vi "SCMP FITS - Make Single FITS Header coop.vi"(6 "FITS info":T1={"File name"="lsob_demo_0530_LM_20190529_124525_live_C1_00020_001_lev0.0.fits", "Date"="2019-05-29T12:45:25"}, 7 "Camera.lvclass":refnum<class "Camera.lvclass">, 8 "error in":errorcluster, 9 "NAXIS":string="2", 10 "FITS Header":T2={"Wavelength (nm)"=530.15, "Exposure (s)"=0.05, "Tuning Delay (ms)"=1000.0, "Beam Type (-1/1)"=1.0, "Tuning Voltages"=[1.111, 2.222, 3.333, 4.444], "Observer"="observer", "Light Shapping Diffuser"=enum."In Beam", "Comment"="", "Data Type"=enum."HOLE", "Mod Cycles"=0, "SCD Calibration Optics"=enum."1 - Polarizer @0, I+Q", "SCD Emission Line Filter"=enum."1-557.6nm", "Cookbook"="", "COMP-S Calibration Wheel"=enum."Dark", "COMP-S Andover Filter Wheel"=enum."530.3nm/HWB 0.34nm (Fe XIV)", "FOV Rotation (deg)"=66.0, "Objective Lens Position (mm)"=0.0, "Occulter size"=0.0, "Time End"=timestamp(3382374145.421875 s since 1904-01-01), "Acc Exposure (s)"=0.0, "Time Stamp Array"=[], "Camera Serial Number"=[], "Camera Temp"=[], "Camera PI (mm)"=[], "Time Start"=timestamp(3382374145.421875 s since 1904-01-01), "Peripherals"={"ILX controler"=FALSE, "Zone temperatures"=FALSE, "Andor"=FALSE, "Andor 2"=FALSE, "PI Stages"=FALSE, "AISAS mechanisms"=FALSE, "AISAS Mech.lvclass"=refnum, "Zone temp ref"=variant, "FWs"=FALSE}, "FITS paths"=[], "Cameras"=enum."Andor", "load preset cbk"=FALSE, "periodic check count"=0, "COMP-S Calibration Wheel 2"=enum."Dark", "Calib"=enum."Dark", "Abso Aperture"=66.0, "Nominal Aperture"=66.0} {"Nominal Aperture" format="%.1f"; "Abso Aperture" format="%.1f"; "Camera PI (mm)" format="%_3g"; "Acc Exposure (s)" format="%^.3g"; "Occulter size" format="%.2f"; "Objective Lens Position (mm)" min=70.0 max=152.0 format="%.2f"; "FOV Rotation (deg)" format="%.1f"; "Exposure (s)" format="%^.3g"; "Wavelength (nm)" format="%_6g"}, 11 "Image #":i32) -> (0 "error out":errorcluster, 1 "23040 Byte Header":string="SIMPLE  =                              T / CONFORMS TO FITS STANDARD            BITPIX  =                             32 / BITS PER PIXEL                       NAXIS   =                              2 / DATA DIMENSIONS IN FITS FILE         NAXIS1  =                              0 / XDIM (PIXELS)                        NAXIS2  =                              0 / YDIM (PIXELS)                        NAXIS3  =                              4 / 4 POLARIZATION STATES                NAXIS4  =                              1 / 1 CAMERA                             ORIGIN  =                        'AISAS' / SCIENTIFIC GROUP                     OBSERVER=                     'SCHWARTZ' / NAME OF OBSERVER                     TELESCOP=                   '20CM ZEISS' / NAME OF TELESCOPE                    LOCATION=            'LOMNICKY PEAK OBS' / LOCATION OF TELESCOPE                INSTRUME=                          'SCD' / NAME OF INSTRUMENT                   BZERO   =                             0. /  ADU OFFSET                          FOCUS   =                             26 / CAMERA-STAGE POSITION (MM)           ROTPOS  =                           66.0 / ROTATIONAL POSITION (DEG)            DIFFUSER=                      'IN BEAM' / 0=IN BEAM, 1=OUT OF BEAM             FW-WVLNG=                        '557.6' / PRE-FILTER CENTER WAVELENGTH (NM)    FW-CALIB=                         'DARK' / CAL-WHEEL POSITION                   CAM-SN1 =                    'SCC-02209' / CAMERA SERIAL NUMBER                 CAM-TEMP=                       0.000000 / FOCAL PLANE TEMP (C)                 TUNEDLAY=                           1000 / LCVR RELAXATION DELAY (mS)           DATE_OBS=                     '3/7/2011' / DATE OF OBSERVATION START (UTC)      TIME_OBS=                   '212225.421' / TIME OF OBSERVATION (UTC)            EXPOSURE=                       0.050000 / EXPOSURE TIME (S)                    MODC    =                              0 / NUMBER OF IMAGES AT EACH STATE       NLC-1   =                          1.111 / TUNING VOLTAGE-1                     NLC-2   =                          2.222 / TUNING VOLTAGE-2                     NLC-3   =                          3.333 / TUNING VOLTAGE-3                     NLC-4   =                          4.444 / TUNING VOLTAGE-4                     NLC-5   =                          0.000 / TUNING VOLTAGE-5                     BEAM    =                              1 / BEAM (0=ON BAND OR 1=CONTINUUM)      WAVELENG=                         530.15 / WAVELENGTH OF OBS (NM)               COMMHEAD=                             '' / OBSERVER COMMENT                     COOKBOOK=                                / COOKBOOK  LOADED                     COMMENT                                                                         COMMENT                                                                         COMMENT                                                                         COMMENT                                                                         COMMENT                                                                         COMMENT                                                                         COMMENT                                                                         COMMENT                                                                         COMMENT                                                                         COMMENT                                                                         COMMENT                                                                         COMMENT                                                                         COMMENT                                                                         COMMENT                                                                         COMMENT                                                                         COMMENT                                                                         COMMENT                                                                         COMMENT                                                                         COMMENT                                                                         COMMENT                                                                         COMMENT                                                                         COMMENT                                                                         COMMENT                                                                         COMMENT                                                                         COMMENT                                                                         COMMENT                                                                         COMMENT                                                                         COMMENT                                                                         COMMENT                                                                         COMMENT                                                                         COMMENT                                                                         COMMENT                                                                         COMMENT                                                                         COMMENT                                                                         COMMENT                                                                         COMMENT                                                                         COMMENT                                                                         COMMENT                                                                         COMMENT                                                                         COMMENT                                                                         COMMENT                                                                         COMMENT                                                                         COMMENT                                                                         COMMENT                                                                         COMMENT                                                                         COMMENT                                                                         COMMENT                                                                         COMMENT                                                                         COMMENT                                                                         COMMENT                                                                         COMMENT                                                                         COMMENT                                                                         COMMENT                                                                         COMMENT                                                                         COMMENT                                                                         COMMENT                                                                         COMMENT                                                                         COMMENT                                                                         COMMENT                                                                         COMMENT                                                                         COMMENT                                                                         COMMENT                                                                         COMMENT                                                                         COMMENT                                                                         COMMENT                                                                         COMMENT                                                                         COMMENT                                                                         COMMENT                                                                         COMMENT                                                                         COMMENT                                                                         COMMENT                                                                         COMMENT                                                                         COMMENT                                                                         COMMENT                                                                         COMMENT                                                                         COMMENT                                                                         COMMENT                                                                         COMMENT                                                                         COMMENT                                                                         COMMENT                                                                         COMMENT                                                                         COMMENT                                                                         COMMENT                                                                         COMMENT                                                                         COMMENT                                                                         COMMENT                                                                         COMMENT                                                                         COMMENT                                                                         COMMENT                                                                         COMMENT                                                                         COMMENT                                                                         COMMENT                                                                         COMMENT                                                                         COMMENT                                                                         COMMENT                                                                         COMMENT                                                                         COMMENT                                                                         COMMENT                                                                         COMMENT                                                                         COMMENT                                                                         COMMENT                                                                         COMMENT                                                                         COMMENT                                                                         COMMENT                                                                         COMMENT                                                                         COMMENT                                                                         COMMENT                                                                         COMMENT                                                                         COMMENT                                                                         COMMENT                                                                         COMMENT                                                                         COMMENT                                                                         COMMENT                                                                         COMMENT                                                                         COMMENT                                                                         COMMENT                                                                         COMMENT                                                                         COMMENT                                                                         COMMENT                                                                         COMMENT                                                                         COMMENT                                                                         COMMENT                                                                         COMMENT                                                                         COMMENT                                                                         COMMENT                                                                         COMMENT                                                                         COMMENT                                                                         COMMENT                                                                         COMMENT                                                                         COMMENT                                                                         COMMENT                                                                         COMMENT                                                                         COMMENT                                                                         COMMENT                                                                         COMMENT                                                                         COMMENT                                                                         COMMENT                                                                         COMMENT                                                                         COMMENT                                                                         COMMENT                                                                         COMMENT                                                                         COMMENT                                                                         COMMENT                                                                         COMMENT                                                                         COMMENT                                                                         COMMENT                                                                         COMMENT                                                                         COMMENT                                                                         COMMENT                                                                         COMMENT                                                                         COMMENT                                                                         COMMENT                                                                         COMMENT                                                                         COMMENT                                                                         COMMENT                                                                         COMMENT                                                                         COMMENT                                                                         COMMENT                                                                         COMMENT                                                                         COMMENT                                                                         COMMENT                                                                         COMMENT                                                                         COMMENT                                                                         COMMENT                                                                         COMMENT                                                                         COMMENT                                                                         COMMENT                                                                         COMMENT                                                                         COMMENT                                                                         COMMENT                                                                         COMMENT                                                                         COMMENT                                                                         COMMENT                                                                         COMMENT                                                                         COMMENT                                                                         COMMENT                                                                         COMMENT                                                                         COMMENT                                                                         COMMENT                                                                         COMMENT                                                                         COMMENT                                                                         COMMENT                                                                         COMMENT                                                                         COMMENT                                                                         COMMENT                                                                         COMMENT                                                                         COMMENT                                                                         COMMENT                                                                         COMMENT                                                                         COMMENT                                                                         COMMENT                                                                         COMMENT                                                                         COMMENT                                                                         COMMENT                                                                         COMMENT                                                                         COMMENT                                                                         COMMENT                                                                         COMMENT                                                                         COMMENT                                                                         COMMENT                                                                         COMMENT                                                                         COMMENT                                                                         COMMENT                                                                         COMMENT                                                                         COMMENT                                                                         COMMENT                                                                         COMMENT                                                                         COMMENT                                                                         COMMENT                                                                         COMMENT                                                                         COMMENT                                                                         COMMENT                                                                         COMMENT                                                                         COMMENT                                                                         COMMENT                                                                         COMMENT                                                                         COMMENT                                                                         COMMENT                                                                         COMMENT                                                                         COMMENT                                                                         COMMENT                                                                         COMMENT                                                                         COMMENT                                                                         COMMENT                                                                         COMMENT                                                                         COMMENT                                                                         COMMENT                                                                         COMMENT                                                                         COMMENT                                                                         COMMENT                                                                         COMMENT                                                                         COMMENT                                                                         COMMENT                                                                         COMMENT                                                                         COMMENT                                                                         COMMENT                                                                         COMMENT                                                                         COMMENT                                                                         COMMENT                                                                         COMMENT                                                                         COMMENT                                                                         COMMENT                                                                         COMMENT                                                                         COMMENT                                                                         COMMENT                                                                         COMMENT                                                                         COMMENT                                                                         COMMENT                                                                         COMMENT                                                                         COMMENT                                                                         COMMENT                                                                         COMMENT                                                                         COMMENT                                                                         END                                                                             ", 3 "final header byte length":i32=23040)   [LabVIEW 2014]
uses:
  Controls/SCD - FITS Cluster.ctl
  AISAS/Mech/AISAS Mech.lvclass
  AISAS/Controls/Diffuser.ctl
  Controls/FITS Data type.ctl
  Controls/SCD - Calibration Optics Filter Wheel.ctl
  Controls/SCD - EDT - Emission Line Filter Wheel.ctl
  Controls/CoMP-S Controls/Polarization Optics Filter Wheel.ctl
  Controls/CoMP-S Controls/Emission Line Filter Wheel.ctl
  AISAS/Controls/focus.ctl
  Controls/peripherals.ctl
  Controls/Cameras select.ctl
  Controls/Fits info.ctl
  Camera/Camera/Camera.lvclass
  Controls/Globals.vi
panel:
  out "Required COMMENT Rows":i32
  in  "NAXIS2":string="2160"
  in  "NAXIS1":string="2560"
  out "Header Rows":i32=34
  out "FITS Header":string[](array[string])=["SIMPLE  =                              T / CONFORMS TO FITS STANDARD            ", "BITPIX  =                             32 / BITS PER PIXEL                       ", "NAXIS   =                              2 / DATA DIMENSIONS IN FITS FILE         ", "NAXIS1  =                              0 / XDIM (PIXELS)                        ", "NAXIS2  =                              0 / YDIM (PIXELS)                        ", "NAXIS3  =                              4 / 4 POLARIZATION STATES                ", "NAXIS4  =                              1 / 1 CAMERA                             ", "ORIGIN  =                        'AISAS' / SCIENTIFIC GROUP                     ", "OBSERVER=                     'SCHWARTZ' / NAME OF OBSERVER                     ", "TELESCOP=                   '20CM ZEISS' / NAME OF TELESCOPE                    ", "LOCATION=            'LOMNICKY PEAK OBS' / LOCATION OF TELESCOPE                ", "INSTRUME=                          'SCD' / NAME OF INSTRUMENT                   ", "BZERO   =                             0. /  ADU OFFSET                          ", "FOCUS   =                             26 / CAMERA-STAGE POSITION (MM)           ", "ROTPOS  =                           66.0 / ROTATIONAL POSITION (DEG)            ", "DIFFUSER=                      'IN BEAM' / 0=IN BEAM, 1=OUT OF BEAM             ", "FW-WVLNG=                        '557.6' / PRE-FILTER CENTER WAVELENGTH (NM)    ", "FW-CALIB=                         'DARK' / CAL-WHEEL POSITION                   ", "CAM-SN1 =                    'SCC-02209' / CAMERA SERIAL NUMBER                 ", "CAM-TEMP=                       0.000000 / FOCAL PLANE TEMP (C)                 ", "TUNEDLAY=                           1000 / LCVR RELAXATION DELAY (mS)           ", "DATE_OBS=                     '3/7/2011' / DATE OF OBSERVATION START (UTC)      ", "TIME_OBS=                   '212225.421' / TIME OF OBSERVATION (UTC)            ", "EXPOSURE=                       0.050000 / EXPOSURE TIME (S)                    ", "MODC    =                              0 / NUMBER OF IMAGES AT EACH STATE       ", "NLC-1   =                          1.111 / TUNING VOLTAGE-1                     ", "NLC-2   =                          2.222 / TUNING VOLTAGE-2                     ", "NLC-3   =                          3.333 / TUNING VOLTAGE-3                     ", "NLC-4   =                          4.444 / TUNING VOLTAGE-4                     ", "NLC-5   =                          0.000 / TUNING VOLTAGE-5                     ", "BEAM    =                              1 / BEAM (0=ON BAND OR 1=CONTINUUM)      ", "WAVELENG=                         530.15 / WAVELENGTH OF OBS (NM)               ", "COMMHEAD=                             '' / OBSERVER COMMENT                     ", "COOKBOOK=                                / COOKBOOK  LOADED                     ", "COMMENT                                                                         ", "COMMENT                                                                         ", "COMMENT                                                                         ", "COMMENT                                                                         ", "COMMENT                                                                         ", "COMMENT                                                                         ", "COMMENT                                                                         ", "COMMENT                                                                         ", "COMMENT                                                                         ", "COMMENT                                                                         ", "COMMENT                                                                         ", "COMMENT                                                                         ", "COMMENT                                                                         ", "COMMENT                                                                         ", "COMMENT                                                                         ", "COMMENT                                                                         ", "COMMENT                                                                         ", "COMMENT                                                                         ", "COMMENT                                                                         ", "COMMENT                                                                         ", "COMMENT                                                                         ", "COMMENT                                                                         ", "COMMENT                                                                         ", "COMMENT                                                                         ", "COMMENT                                                                         ", "COMMENT                                                                         ", "COMMENT                                                                         ", "COMMENT                                                                         ", "COMMENT                                                                         ", "COMMENT                                                                         ", "COMMENT                                                                         ", "COMMENT                                                                         ", "COMMENT                                                                         ", "COMMENT                                                                         ", "COMMENT                                                                         ", "COMMENT                                                                         ", "COMMENT                                                                         ", "COMMENT                                                                         ", "COMMENT                                                                         ", "COMMENT                                                                         ", "COMMENT                                                                         ", "COMMENT                                                                         ", "COMMENT                                                                         ", "COMMENT                                                                         ", "COMMENT                                                                         ", "COMMENT                                                                         ", "COMMENT                                                                         ", "COMMENT                                                                         ", "COMMENT                                                                         ", "COMMENT                                                                         ", "COMMENT                                                                         ", "COMMENT                                                                         ", "COMMENT                                                                         ", "COMMENT                                                                         ", "COMMENT                                                                         ", "COMMENT                                                                         ", "COMMENT                                                                         ", "COMMENT                                                                         ", "COMMENT                                                                         ", "COMMENT                                                                         ", "COMMENT                                                                         ", "COMMENT                                                                         ", "COMMENT                                                                         ", "COMMENT                                                                         ", "COMMENT                                                                         ", "COMMENT                                                                         ", "COMMENT                                                                         ", "COMMENT                                                                         ", "COMMENT                                                                         ", "COMMENT                                                                         ", "COMMENT                                                                         ", "COMMENT                                                                         ", "COMMENT                                                                         ", "COMMENT                                                                         ", "COMMENT                                                                         ", "COMMENT                                                                         ", "COMMENT                                                                         ", "COMMENT                                                                         ", "COMMENT                                                                         ", "COMMENT                                                                         ", "COMMENT                                                                         ", "COMMENT                                                                         ", "COMMENT                                                                         ", "COMMENT                                                                         ", "COMMENT                                                                         ", "COMMENT                                                                         ", "COMMENT                                                                         ", "COMMENT                                                                         ", "COMMENT                                                                         ", "COMMENT                                                                         ", "COMMENT                                                                         ", "COMMENT                                                                         ", "COMMENT                                                                         ", "COMMENT                                                                         ", "COMMENT                                                                         ", "COMMENT                                                                         ", "COMMENT                                                                         ", "COMMENT                                                                         ", "COMMENT                                                                         ", "COMMENT                                                                         ", "COMMENT                                                                         ", "COMMENT                                                                         ", "COMMENT                                                                         ", "COMMENT                                                                         ", "COMMENT                                                                         ", "COMMENT                                                                         ", "COMMENT                                                                         ", "COMMENT                                                                         ", "COMMENT                                                                         ", "COMMENT                                                                         ", "COMMENT                                                                         ", "COMMENT                                                                         ", "COMMENT                                                                         ", "COMMENT                                                                         ", "COMMENT                                                                         ", "COMMENT                                                                         ", "COMMENT                                                                         ", "COMMENT                                                                         ", "COMMENT                                                                         ", "COMMENT                                                                         ", "COMMENT                                                                         ", "COMMENT                                                                         ", "COMMENT                                                                         ", "COMMENT                                                                         ", "COMMENT                                                                         ", "COMMENT                                                                         ", "COMMENT                                                                         ", "COMMENT                                                                         ", "COMMENT                                                                         ", "COMMENT                                                                         ", "COMMENT                                                                         ", "COMMENT                                                                         ", "COMMENT                                                                         ", "COMMENT                                                                         ", "COMMENT                                                                         ", "COMMENT                                                                         ", "COMMENT                                                                         ", "COMMENT                                                                         ", "COMMENT                                                                         ", "COMMENT                                                                         ", "COMMENT                                                                         ", "COMMENT                                                                         ", "COMMENT                                                                         ", "COMMENT                                                                         ", "COMMENT                                                                         ", "COMMENT                                                                         ", "COMMENT                                                                         ", "COMMENT                                                                         ", "COMMENT                                                                         ", "COMMENT                                                                         ", "COMMENT                                                                         ", "COMMENT                                                                         ", "COMMENT                                                                         ", "COMMENT                                                                         ", "COMMENT                                                                         ", "COMMENT                                                                         ", "COMMENT                                                                         ", "COMMENT                                                                         ", "COMMENT                                                                         ", "COMMENT                                                                         ", "COMMENT                                                                         ", "COMMENT                                                                         ", "COMMENT                                                                         ", "COMMENT                                                                         ", "COMMENT                                                                         ", "COMMENT                                                                         ", "COMMENT                                                                         ", "COMMENT                                                                         ", "COMMENT                                                                         ", "COMMENT                                                                         ", "COMMENT                                                                         ", "COMMENT                                                                         ", "COMMENT                                                                         ", "COMMENT                                                                         ", "COMMENT                                                                         ", "COMMENT                                                                         ", "COMMENT                                                                         ", "COMMENT                                                                         ", "COMMENT                                                                         ", "COMMENT                                                                         ", "COMMENT                                                                         ", "COMMENT                                                                         ", "COMMENT                                                                         ", "COMMENT                                                                         ", "COMMENT                                                                         ", "COMMENT                                                                         ", "COMMENT                                                                         ", "COMMENT                                                                         ", "COMMENT                                                                         ", "COMMENT                                                                         ", "COMMENT                                                                         ", "COMMENT                                                                         ", "COMMENT                                                                         ", "COMMENT                                                                         ", "COMMENT                                                                         ", "COMMENT                                                                         ", "COMMENT                                                                         ", "COMMENT                                                                         ", "COMMENT                                                                         ", "COMMENT                                                                         ", "COMMENT                                                                         ", "COMMENT                                                                         ", "COMMENT                                                                         ", "COMMENT                                                                         ", "COMMENT                                                                         ", "COMMENT                                                                         ", "COMMENT                                                                         ", "COMMENT                                                                         ", "COMMENT                                                                         ", "COMMENT                                                                         ", "COMMENT                                                                         ", "COMMENT                                                                         ", "COMMENT                                                                         ", "COMMENT                                                                         ", "COMMENT                                                                         ", "COMMENT                                                                         ", "COMMENT                                                                         ", "COMMENT                                                                         ", "COMMENT                                                                         ", "COMMENT                                                                         ", "COMMENT                                                                         ", "COMMENT                                                                         ", "COMMENT                                                                         ", "COMMENT                                                                         ", "COMMENT                                                                         ", "COMMENT                                                                         ", "COMMENT                                                                         ", "COMMENT                                                                         ", "COMMENT                                                                         ", "COMMENT                                                                         ", "COMMENT                                                                         ", "COMMENT                                                                         ", "COMMENT                                                                         ", "COMMENT                                                                         ", "COMMENT                                                                         ", "COMMENT                                                                         ", "COMMENT                                                                         ", "COMMENT                                                                         ", "COMMENT                                                                         ", "COMMENT                                                                         ", "COMMENT                                                                         ", "COMMENT                                                                         ", "COMMENT                                                                         ", "COMMENT                                                                         ", "COMMENT                                                                         ", "COMMENT                                                                         ", "COMMENT                                                                         ", "COMMENT                                                                         ", "COMMENT                                                                         ", "COMMENT                                                                         ", "COMMENT                                                                         ", "COMMENT                                                                         ", "COMMENT                                                                         ", "END                                                                             "]
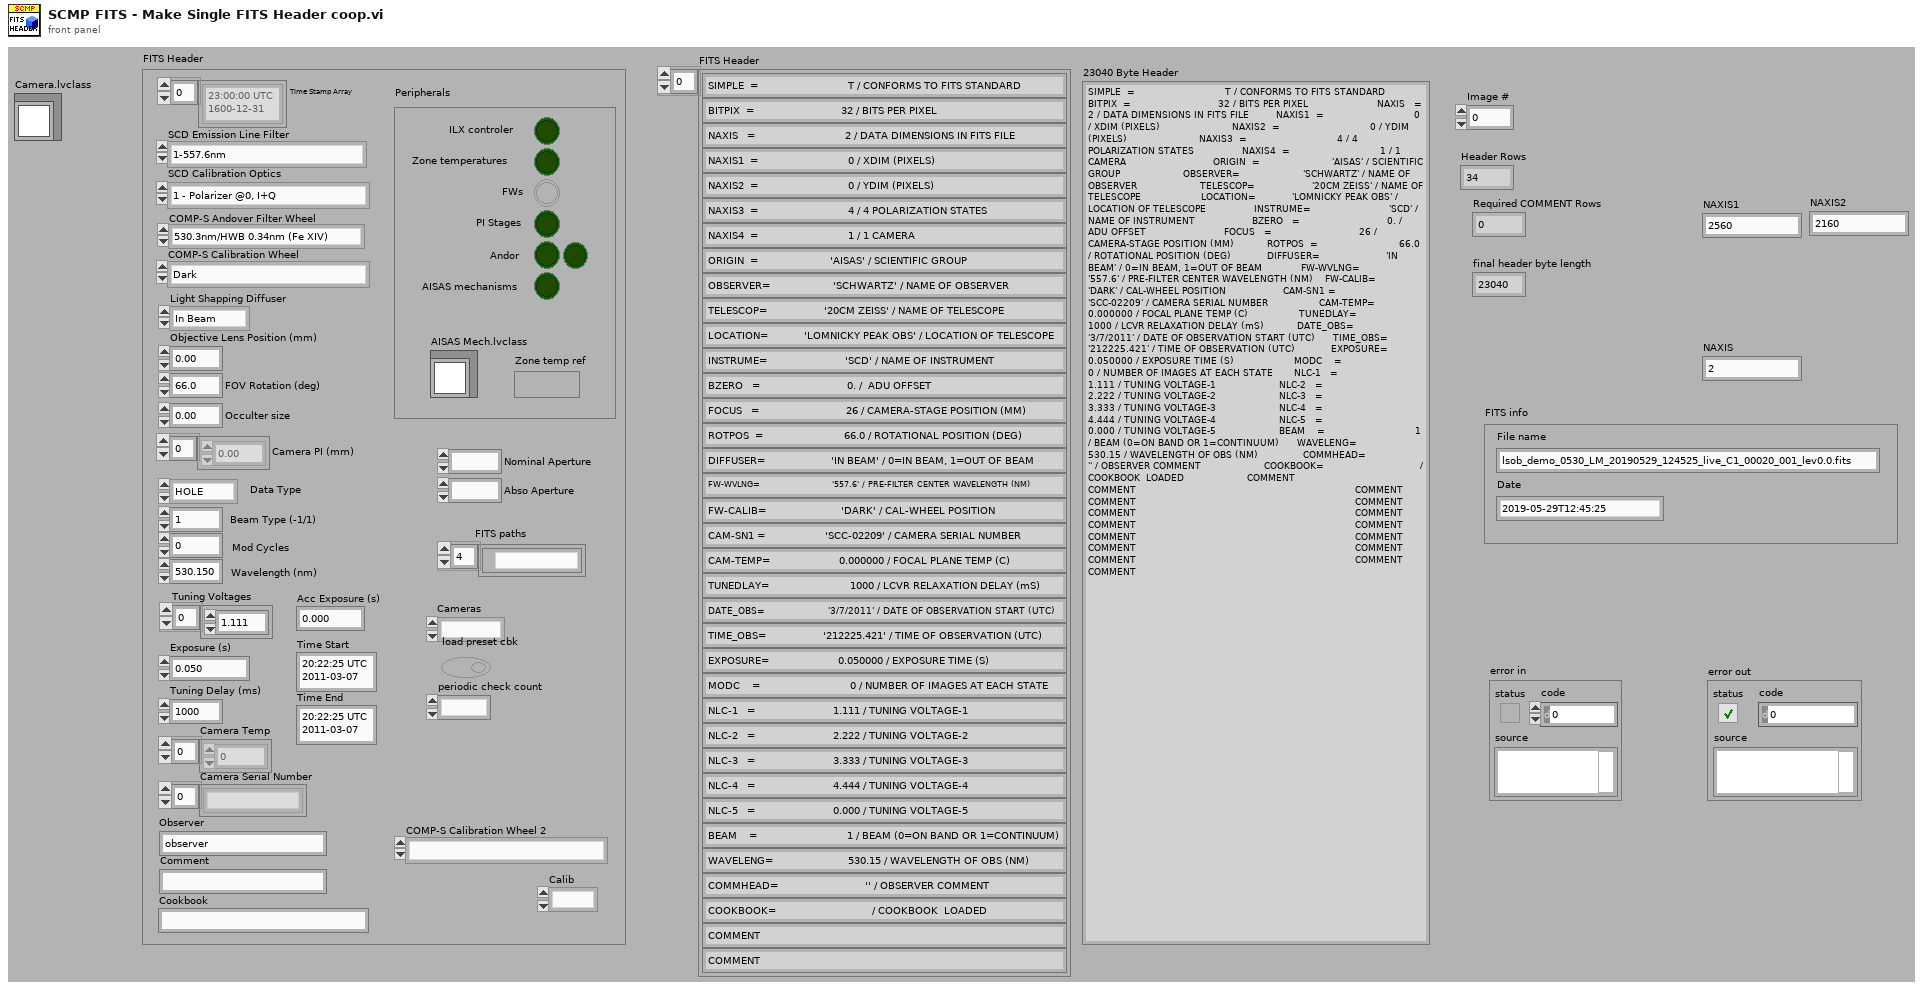
[diagram p1: front panel]
types:
  T1 = typedef "Fits info.ctl" = cluster{"File name":string, "Date":string}
  T2 = typedef "SCD - FITS Cluster.ctl" = cluster{"Wavelength (nm)":dbl, "Exposure (s)":dbl, "Tuning Delay (ms)":dbl, "Beam Type (-1/1)":dbl, "Tuning Voltages":dbl[], "Observer":string, "Light Shapping Diffuser":T3, "Comment":string, "Data Type":T4, "Mod Cycles":u16, "SCD Calibration Optics":T5, "SCD Emission Line Filter":T6, "Cookbook":string, "COMP-S Calibration Wheel":T7, "COMP-S Andover Filter Wheel":T8, "FOV Rotation (deg)":dbl, "Objective Lens Position (mm)":T9, "Occulter size":dbl, "Time End":timestamp, "Acc Exposure (s)":dbl, "Time Stamp Array":timestamp[], "Camera Serial Number":string[], "Camera Temp":dbl[], "Camera PI (mm)":dbl[], "Time Start":timestamp, "Peripherals":T10, "FITS paths":path[], "Cameras":T11, "load preset cbk":bool, "periodic check count":i32, "COMP-S Calibration Wheel 2":T7, "Calib":enum16{"Dark", "Flat"}, "Abso Aperture":dbl, "Nominal Aperture":dbl}
  T3 = typedef "Diffuser.ctl" = enum16{"Out of Beam", "In Beam"}
  T4 = typedef "FITS Data type.ctl" = enum16{"LIVE", "DARK", "FLAT", "CALI", "OBSE", "ABSO", "AURE", "TARG", "OBJE", "HOLE", "OREX", "THRO", "CHIP"}
  T5 = typedef "SCD - Calibration Optics Filter Wheel.ctl" = enum16{"1 - Polarizer @0, I+Q", "2 - Polarizer @90, I-Q", "3 - Polarizer @45, I+U", "4 - Polarizer @135, I-U", "5 - Polarizer @0, Retarder @45, I+V", "6 - Polarizer @0, Retarder @135, I-V", "7 - Dark", "8 - Clear", "9 - N/A"}
  T6 = typedef "SCD - EDT - Emission Line Filter Wheel.ctl" = enum16{"1-557.6nm", "2-587.6nm", "3-589.6nm", "4-630.2nm", "5-656.4nm", "6-849.8nm", "7-854.2nm", "8-866.2nm", "9-1083.0nm"}
  T7 = typedef "Polarization Optics Filter Wheel.ctl" = enum16{"Dark", "Clear", "Exchange Lens", "Polarizer @0, I+Q", "Polarizer @90, I-Q", "Polarizer @45, I+U", "Polarizer @135, I-U", "Polarizer @0, Retarder @45, I+V", "Polarizer @0, Retarder @135, I-V"}
  T8 = typedef "Emission Line Filter Wheel.ctl" = enum16{"530.3nm/HWB 0.34nm (Fe XIV)", "587.6nm/HBW 0.44nm (He I D3)", "637.5nm/HBW 0.53nm (Fe X)", "656.3nm/HBW 0.57nm (H-Alpha)", "789.2nm/HBW 0.85nm (Fe XI)", "854.2nm/HBW 1.01nm (Ca I)", "1074.7nm/HBW 2.34nm (Fe XIII)", "1079.8nm/HBW 1.64nm (Fe XIII)", "1083.0nm/HBW 1.66nm (He I)"}
  T9 = typedef "focus.ctl" = dbl
  T10 = typedef "peripherals.ctl" = cluster{"ILX controler":bool, "Zone temperatures":bool, "Andor":bool, "Andor 2":bool, "PI Stages":bool, "AISAS mechanisms":bool, "AISAS Mech.lvclass":refnum<class "AISAS Mech.lvclass">, "Zone temp ref":variant, "FWs":bool}
  T11 = typedef "Cameras select.ctl" = enum16{"Andor", "GDR"}
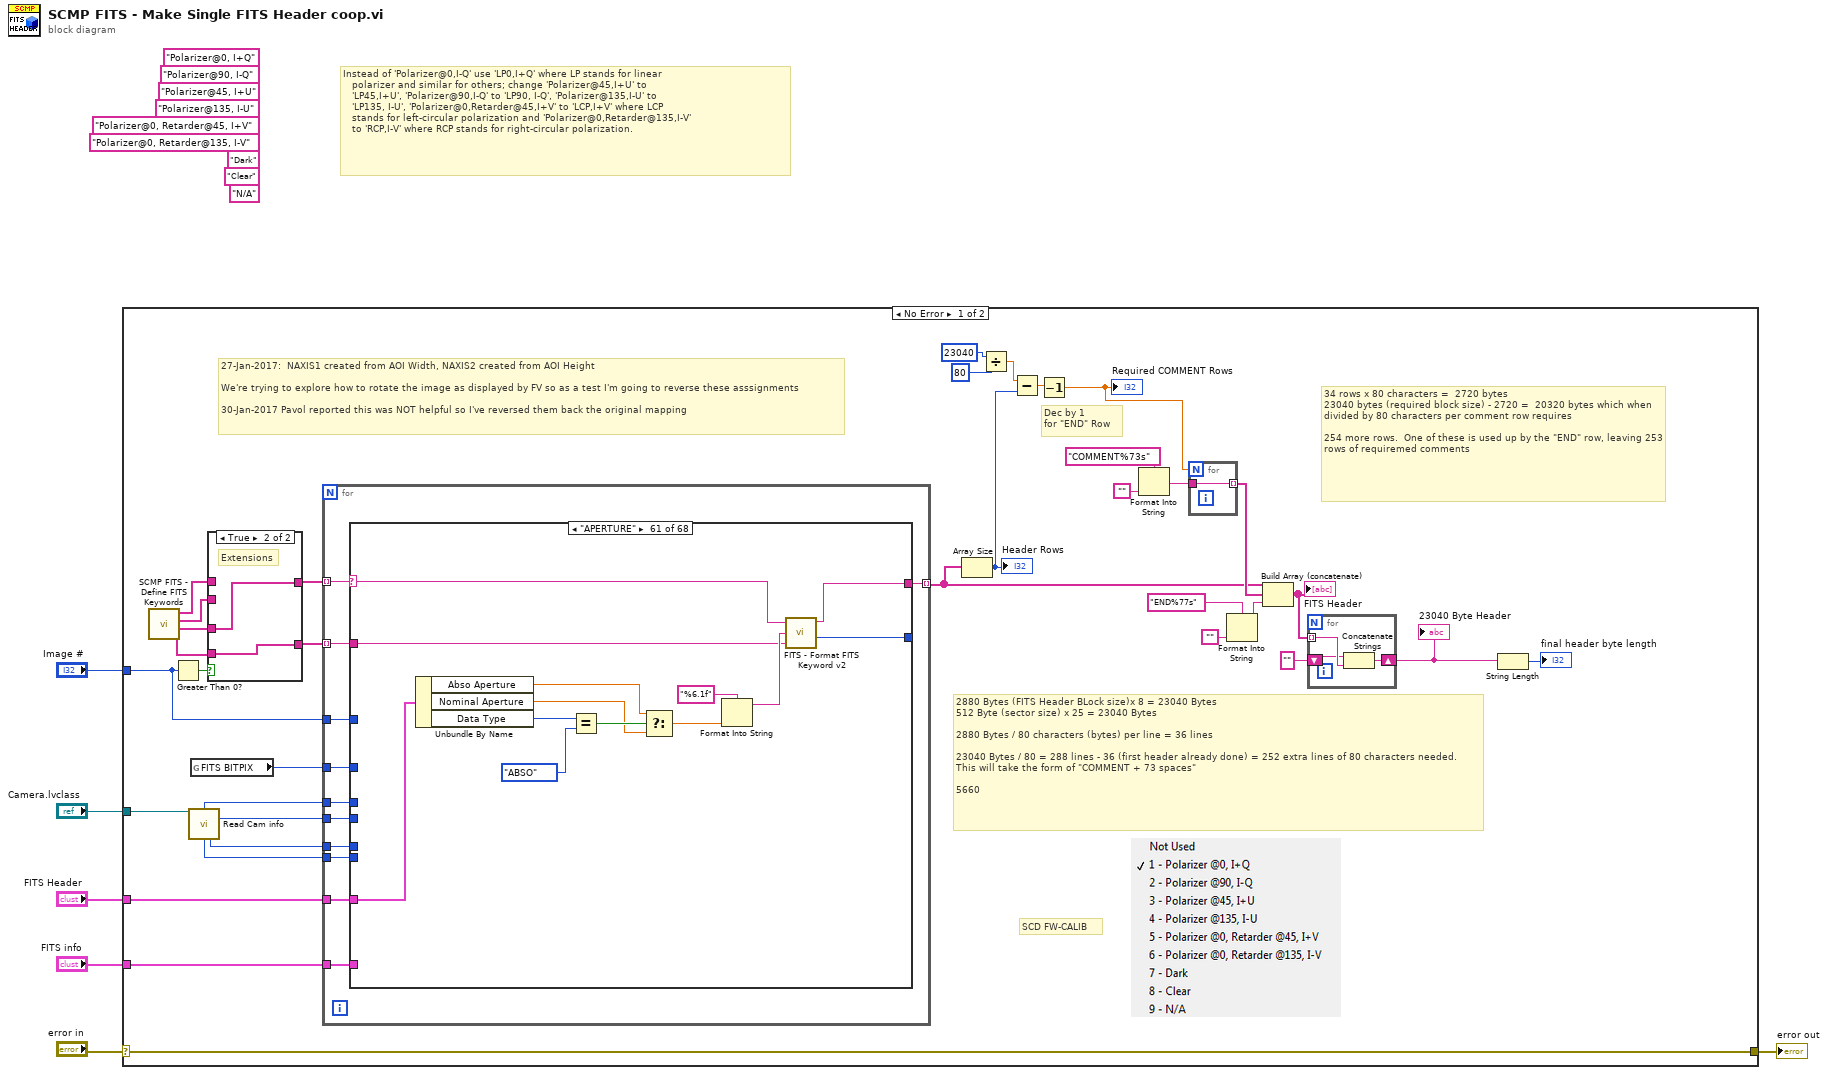
[diagram p0: block diagram]
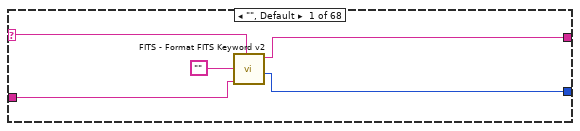
[diagram p3: hidden frame]
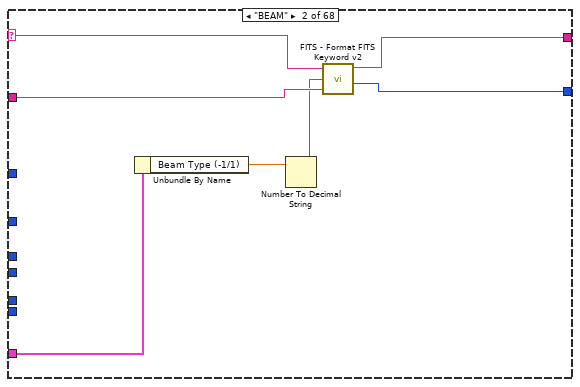
[diagram p4: hidden frame]
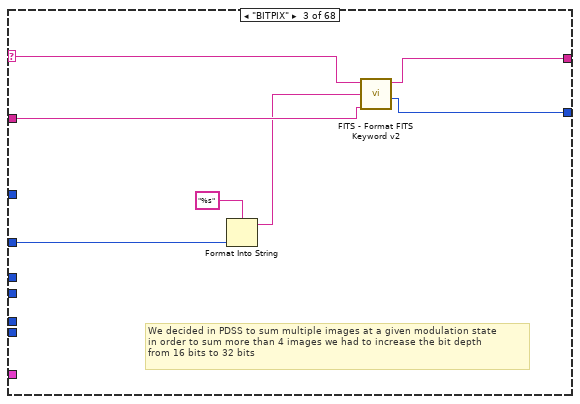
[diagram p5: hidden frame]
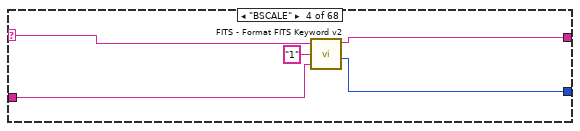
[diagram p6: hidden frame]
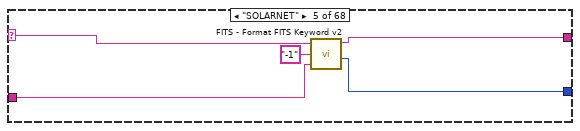
[diagram p7: hidden frame]
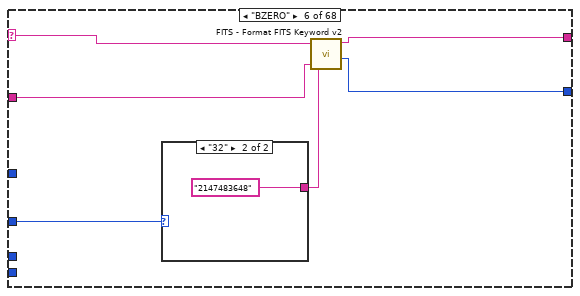
[diagram p8: hidden frame]
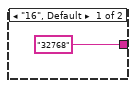
[diagram p9: hidden frame]
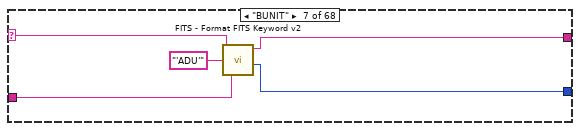
[diagram p10: hidden frame]
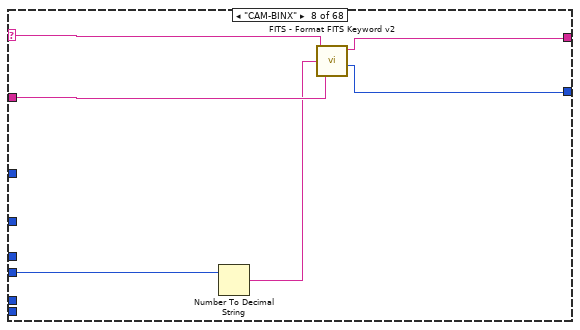
[diagram p11: hidden frame]
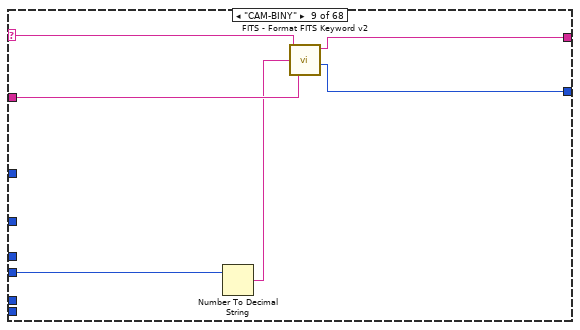
[diagram p12: hidden frame]
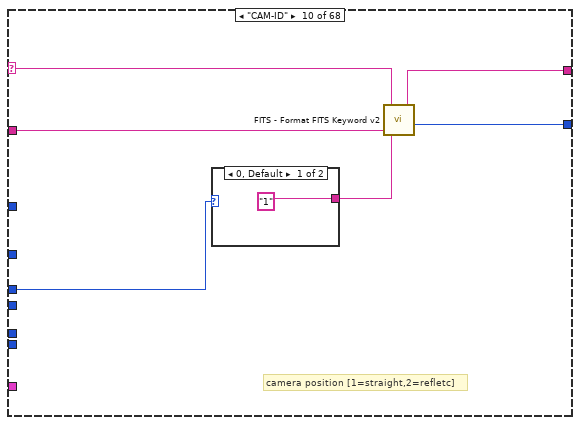
[diagram p13: hidden frame]
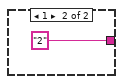
[diagram p14: hidden frame]
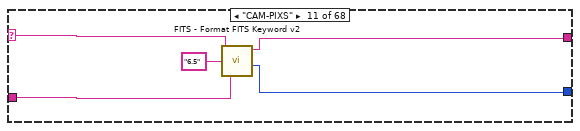
[diagram p15: hidden frame]
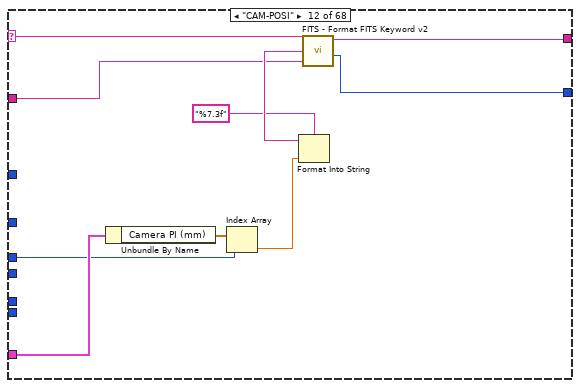
[diagram p16: hidden frame]
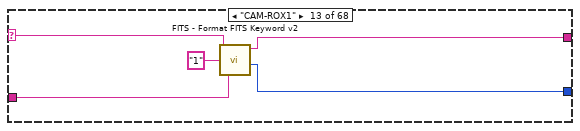
[diagram p17: hidden frame]
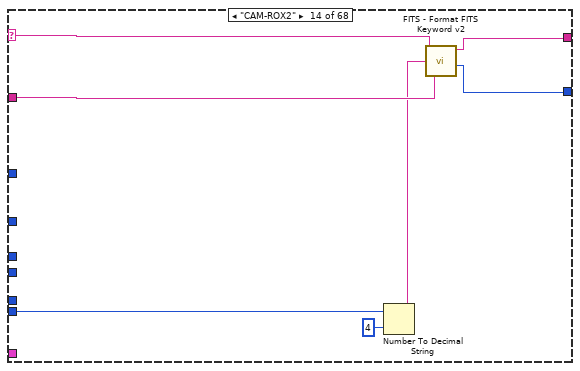
[diagram p18: hidden frame]
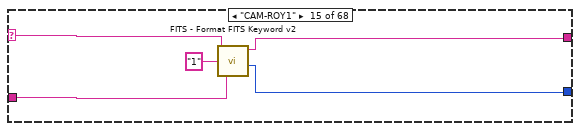
[diagram p19: hidden frame]
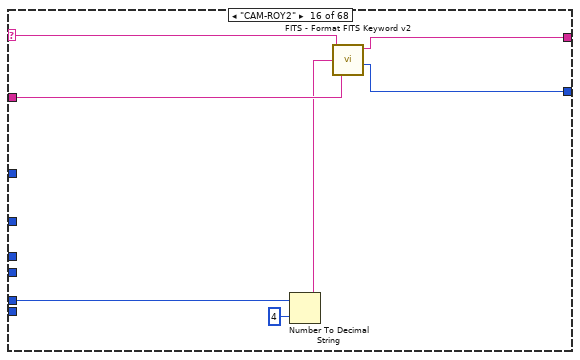
[diagram p20: hidden frame]
diagram:
  (unwired) "N/A" ("element")
  (unwired) "Clear" ("element")
  (unwired) "Dark" ("element")
  (unwired) "Polarizer@0, Retarder@135, I-V" ("element")
  (unwired) "Polarizer@0, Retarder@45, I+V" ("element")
  (unwired) "Polarizer@135, I-U" ("element")
  (unwired) "Polarizer@45, I+U"
  (unwired) "Polarizer@90, I-Q"
  (unwired) "Polarizer@0, I+Q"
  # "Instead of 'Polarizer@0,I-Q' use 'LP0,I+Q' where LP stands for linear\n   polarizer and similar for others; change 'Polarizer@45,I+U' to\n   'LP45,I+U', 'Polarizer@90,I-Q' to 'LP90, I-Q', 'Polarizer@135,I-U' to\n   'LP135, I-U', 'Polarizer@0,Retarder@45,I+V' to 'LCP,I+V' where LCP\n   stands for left-circular polarization and 'Polarizer@0,Retarder@135,I-V'\n   to 'RCP,I-V' where RCP stands for right-circular polarization."
  n1 = case shown="No Error" "error in" {
    selector: "error in" -> [w23 w622]
    tunnel: [w23 w622] -> w5
    tunnel: "Image #" -> [w14 _]
    tunnel: "Camera.lvclass" -> [w12 _]
    tunnel: "FITS Header" -> [w8 _]
    tunnel: "FITS info" -> [w7 _]
    frame No Error {
      # "SCD FW-CALIB"
      # "27-Jan-2017:  NAXIS1 created from AOI Width, NAXIS2 created from AOI Height\n\nWe're trying to explore how to rotate the image as displayed by FV so as a test I'm going to reverse these asssignments\n\n30-Jan-2017 Pavol reported this was NOT helpful so I've reversed them back the original mapping"
      # "34 rows x 80 characters =  2720 bytes\n23040 bytes (required block size) - 2720 =  20320 bytes which when divided by 80 characters per comment row requires\n\n254 more rows.  One of these is used up by the \"END\" row, leaving 253 rows of requiremed comments"
      # "Dec by 1\nfor \"END\" Row"
      # "2880 Bytes (FITS Header BLock size)x 8 = 23040 Bytes\n512 Byte (sector size) x 25 = 23040 Bytes\n\n2880 Bytes / 80 characters (bytes) per line = 36 lines\n\n23040 Bytes / 80 = 288 lines - 36 (first header already done) = 252 extra lines of 80 characters needed.\nThis will take the form of \"COMMENT + 73 spaces\" \n\n5660"
      n2 = call "SCMP FITS - Define FITS Keywords.vi"() -> ("Extension Comments"=w34:string[], "Extension  Keywords"=w35:string[], "Primary Comments"=w36:string[], "Primary Keywords"=w33:string[])  [unwired: 5 in, 3 out]
      n3 = Greater Than 0?(x=w14) -> (x > 0?=w39:bool)
      n4 = call-dynamic "Read Cam info.vi"("Camera in"=w12) -> ("Idx"=w11:i32, "BDiv"=w13:u8, "AOI Width"=w10:i32, "AOI Height"=w9:i32)  [unwired: 5 in, 6 out]
      n5 = global read "Globals.vi" "FITS BITPIX"() -> (w15:enum16{"16", "32"})
      n6 = case shown="True" w39 {
        tunnel: [w47 w49] -> w38
        tunnel: [w46 w48] -> w37
        tunnel: w33 -> [w47 _]
        tunnel: w36 -> [w46 _]
        tunnel: w35 -> [_ w49]
        tunnel: w34 -> [_ w48]
        frame False {
          # "Primary"
        }
        frame True {
          # "Extensions"
        }
      }
      n7 = for {
        tunnel: w38 -> [w56] mode=indexing
        tunnel: w37 -> [w59] mode=indexing
        tunnel: w8 -> [w60]
        tunnel: [w58] -> w22 mode=indexing
        tunnel: w14 -> [w57]
        tunnel: w15 -> [w55]
        tunnel: w7 -> [w54]
        tunnel: w13 -> [w53]
        tunnel: w11 -> [w52]
        tunnel: w10 -> [w51]
        tunnel: w9 -> [w50]
        n8 = case shown="\"APERTURE\"" w56 {
          selector: w56 -> [w65 w72 w79 w84 w89 w95 w101 w108 w114 w120 w126 w135 w141 w149 w153 w161 w171 w181 w187 w194 w202 w226 w233 w248 w260 w266 w274 w284 w295 w306 w316 w321 w329 w334 w341 w345 w353 w362 w394 w399 w404 w411 w415 w422 w430 w449 w456 w467 w472 w482 w492 w502 w512 w522 w530 w538 w545 w551 w556 w560 w574 w582 w587 w591 w597 w608 w613 w620]
          tunnel: w60 -> [_ w69 _ _ _ _ _ _ _ _ _ w130 _ _ _ _ w168 w175 w183 w195 w203 _ w230 w250 w258 w264 w276 w282 _ w303 w313 _ _ _ _ _ w350 w359 w390 _ _ _ _ w419 _ _ _ _ _ w479 w489 w499 w509 w519 w526 w536 w542 _ _ w564 w577 _ _ _ w594 w605 _ w616]
          tunnel: w59 -> [w63 w71 w78 w83 w88 w94 w100 w107 w113 w119 w125 w134 w140 w148 w152 w160 w170 w180 w186 w193 w201 w225 w232 w249 w259 w265 w275 w283 w294 w305 w315 w320 w328 w333 w340 w344 w352 w361 w393 w397 w403 w409 w414 w421 w429 w448 w457 w466 w471 w481 w491 w501 w511 w521 w529 w537 w544 w550 w554 w561 w575 w581 w586 w590 w596 w607 w612 w619]
          tunnel: [w62 w70 w77 w82 w87 w93 w98 w106 w112 w118 w124 w133 w139 w147 w151 w159 w169 w179 w185 w192 w200 w224 w231 w246 w257 w263 w273 w285 w293 w304 w314 w319 w327 w332 w338 w343 w351 w360 w392 w396 w402 w410 w413 w420 w428 w447 w455 w465 w470 w480 w490 w500 w510 w520 w528 w534 w543 w549 w553 w559 w573 w580 w585 w589 w595 w606 w611 w618] -> w58
          tunnel: [w61 w66 w76 w81 w86 w92 w99 w105 w111 w117 w123 w132 w138 w146 w150 w158 w167 w177 w184 w191 w199 w223 w228 w247 w256 w262 w272 w286 w292 w302 w310 w317 w326 w331 w339 w342 w348 w358 w391 w395 w401 w408 w412 w417 w427 w446 w454 w464 w468 w478 w488 w498 w508 w518 w527 w535 w540 w548 w552 w558 w572 w578 w584 w588 w593 w601 w609 w617] -> _
          tunnel: w57 -> [_ _ _ _ _ _ _ _ _ _ _ _ _ _ _ _ _ _ _ _ _ _ _ _ _ _ _ _ _ _ _ _ _ _ _ _ _ _ _ _ _ _ _ _ w425 _ _ _ _ _ _ _ _ _ _ _ _ _ _ _ _ _ _ _ _ _ _ _]
          tunnel: w55 -> [_ _ w75 _ _ w90 _ _ _ _ _ _ _ _ _ _ _ _ _ _ _ _ _ _ _ _ _ _ _ _ _ _ _ _ _ _ _ _ _ _ _ _ _ _ _ _ _ _ _ _ _ _ _ _ _ _ _ _ _ _ _ _ _ _ _ _ _ _]
          tunnel: w54 -> [_ _ _ _ _ _ _ _ _ _ _ _ _ _ _ _ _ _ _ _ _ w221 w227 _ _ _ _ _ _ _ _ _ w325 _ _ _ _ _ _ _ _ _ _ _ _ _ _ _ _ _ _ _ _ _ _ _ _ _ _ _ _ _ _ _ _ _ _ _]
          tunnel: w53 -> [_ _ _ _ _ _ _ w103 w109 _ _ _ _ _ _ _ _ _ _ _ _ _ _ _ _ _ _ _ _ _ _ _ _ _ _ _ _ _ _ _ _ _ _ _ _ _ _ _ _ _ _ _ _ _ _ _ _ _ _ _ _ _ _ _ _ _ _ _]
          tunnel: w52 -> [_ _ _ _ _ _ _ _ _ w115 _ w128 _ _ _ _ w162 w172 _ _ _ _ _ _ _ _ _ _ _ _ _ _ _ _ _ _ _ _ _ _ _ _ _ _ _ _ _ _ _ _ _ _ _ _ _ _ _ _ _ _ _ _ _ _ _ _ _ _]
          tunnel: w51 -> [_ _ _ _ _ _ _ _ _ _ _ _ _ w143 _ _ _ _ _ _ _ _ _ _ _ _ _ _ _ _ _ _ _ _ _ _ _ _ _ _ _ _ _ _ _ w442 w452 _ _ _ _ _ _ _ _ _ _ _ _ _ _ _ _ _ _ _ _ _]
          tunnel: w50 -> [_ _ _ _ _ _ _ _ _ _ _ _ _ _ _ w155 _ _ _ _ _ _ _ _ _ _ _ _ _ _ _ _ _ _ _ _ _ _ _ _ _ _ _ _ _ w441 w453 _ _ _ _ _ _ _ _ _ _ _ _ _ _ _ _ _ _ _ _ _]
          frame "", Default {
            n9 = call "FITS - Format FITS Keyword v2 .vi"("Keyword"=w65, "Value"="", "Comment"=w63) -> ("Formatted fits entry"=w62:string, "Length of line"=w61:i16)  [unwired: 1 in, 1 out]
          }
          frame "BEAM" {
            n10 = Unbundle By Name(w69) -> ("Beam Type (-1/1)"=w67:dbl)
            n11 = Number To Decimal String(number=w67) -> (decimal integer string=w68:string)  [unwired: 1 out]
            n12 = call "FITS - Format FITS Keyword v2 .vi"("Keyword"=w72, "Value"=w68, "Comment"=w71) -> ("Formatted fits entry"=w70:string, "Length of line"=w66:i16)  [unwired: 1 in, 1 out]
          }
          frame "BITPIX" {
            # "We decided in PDSS to sum multiple images at a given modulation state\nin order to sum more than 4 images we had to increase the bit depth\nfrom 16 bits to 32 bits"
            n13 = Format Into String(format string="%s", w75) -> (resulting string=w73:string)  [unwired: 2 in, 1 out]
            n14 = call "FITS - Format FITS Keyword v2 .vi"("Keyword"=w79, "Value"=w73, "Comment"=w78) -> ("Formatted fits entry"=w77:string, "Length of line"=w76:i16)  [unwired: 1 in, 1 out]
          }
          frame "BSCALE" {
            n15 = call "FITS - Format FITS Keyword v2 .vi"("Keyword"=w84, "Value"="1", "Comment"=w83) -> ("Formatted fits entry"=w82:string, "Length of line"=w81:i16)  [unwired: 1 in, 1 out]
          }
          frame "SOLARNET" {
            n16 = call "FITS - Format FITS Keyword v2 .vi"("Keyword"=w89, "Value"="-1", "Comment"=w88) -> ("Formatted fits entry"=w87:string, "Length of line"=w86:i16)  [unwired: 1 in, 1 out]
          }
          frame "BZERO" {
            n17 = case shown="\"32\"" w90 {
              tunnel: ["32768" ("Value") "2147483648" ("Value")] -> w91
              frame "16", Default {
              }
              frame "32" {
              }
            }
            n18 = call "FITS - Format FITS Keyword v2 .vi"("Keyword"=w95, "Value"=w91, "Comment"=w94) -> ("Formatted fits entry"=w93:string, "Length of line"=w92:i16)  [unwired: 1 in, 1 out]
          }
          frame "BUNIT" {
            n19 = call "FITS - Format FITS Keyword v2 .vi"("Keyword"=w101, "Value"="'ADU'", "Comment"=w100) -> ("Formatted fits entry"=w98:string, "Length of line"=w99:i16)  [unwired: 1 in, 1 out]
          }
          frame "CAM-BINX" {
            n20 = Number To Decimal String(number=w103) -> (decimal integer string=w104:string)  [unwired: 1 in]
            n21 = call "FITS - Format FITS Keyword v2 .vi"("Keyword"=w108, "Value"=w104, "Comment"=w107) -> ("Formatted fits entry"=w106:string, "Length of line"=w105:i16)  [unwired: 1 in, 1 out]
          }
          frame "CAM-BINY" {
            n22 = Number To Decimal String(number=w109) -> (decimal integer string=w110:string)  [unwired: 1 in]
            n23 = call "FITS - Format FITS Keyword v2 .vi"("Keyword"=w114, "Value"=w110, "Comment"=w113) -> ("Formatted fits entry"=w112:string, "Length of line"=w111:i16)  [unwired: 1 in, 1 out]
          }
          frame "CAM-ID" {
            # "camera position [1=straight,2=refletc]"
            n24 = case shown="0, Default" w115 {
              tunnel: ["1" ("string") "2" ("string")] -> w116
              frame 0, Default {
              }
              frame 1 {
              }
            }
            n25 = call "FITS - Format FITS Keyword v2 .vi"("Keyword"=w120, "Value"=w116, "Comment"=w119) -> ("Formatted fits entry"=w118:string, "Length of line"=w117:i16)  [unwired: 1 in, 1 out]
          }
          frame "CAM-PIXS" {
            n26 = call "FITS - Format FITS Keyword v2 .vi"("Keyword"=w126, "Value"="6.5", "Comment"=w125) -> ("Formatted fits entry"=w124:string, "Length of line"=w123:i16)  [unwired: 1 in, 1 out]
          }
          frame "CAM-POSI" {
            n27 = Unbundle By Name(w130) -> ("Camera PI (mm)"=w131:dbl[])
            n28 = Index Array(array=w131, index=w128) -> (element=w129:dbl)
            n29 = Format Into String(format string="%7.3f", w129) -> (resulting string=w137:string)  [unwired: 2 in, 1 out]
            n30 = call "FITS - Format FITS Keyword v2 .vi"("Keyword"=w135, "Value"=w137, "Comment"=w134) -> ("Formatted fits entry"=w133:string, "Length of line"=w132:i16)  [unwired: 1 in, 1 out]
          }
          frame "CAM-ROX1" {
            n31 = call "FITS - Format FITS Keyword v2 .vi"("Keyword"=w141, "Value"="1", "Comment"=w140) -> ("Formatted fits entry"=w139:string, "Length of line"=w138:i16)  [unwired: 1 in, 1 out]
          }
          frame "CAM-ROX2" {
            n32 = Number To Decimal String(number=w143, width (-)=i16 4) -> (decimal integer string=w144:string)
            n33 = call "FITS - Format FITS Keyword v2 .vi"("Keyword"=w149, "Value"=w144, "Comment"=w148) -> ("Formatted fits entry"=w147:string, "Length of line"=w146:i16)  [unwired: 1 in, 1 out]
          }
          frame "CAM-ROY1" {
            n34 = call "FITS - Format FITS Keyword v2 .vi"("Keyword"=w153, "Value"="1", "Comment"=w152) -> ("Formatted fits entry"=w151:string, "Length of line"=w150:i16)  [unwired: 1 in, 1 out]
          }
          frame "CAM-ROY2" {
            n35 = Number To Decimal String(number=w155, width (-)=i16 4) -> (decimal integer string=w156:string)
            n36 = call "FITS - Format FITS Keyword v2 .vi"("Keyword"=w161, "Value"=w156, "Comment"=w160) -> ("Formatted fits entry"=w159:string, "Length of line"=w158:i16)  [unwired: 1 in, 1 out]
          }
          frame "CAM-SN" {
            w166 = "'" ("string")
            n37 = Unbundle By Name(w168) -> ("Camera Serial Number"=w164:string[])
            n38 = Index Array(array=w164, index=w162) -> (element=w163:string)
            n39 = Concatenate Strings(w166, w163, w166) -> (w165:string)
            n40 = call "FITS - Format FITS Keyword v2 .vi"("Keyword"=w171, "Value"=w165, "Comment"=w170) -> ("Formatted fits entry"=w169:string, "Length of line"=w167:i16)  [unwired: 1 in, 1 out]
          }
          frame "CAM-TEMP" {
            n41 = Unbundle By Name(w175) -> ("Camera Temp"=w174:dbl[])
            n42 = Index Array(array=w174, index=w172) -> (element=w173:dbl)
            n43 = Format Into String(format string="%6.2f", w173) -> (resulting string=w178:string)  [unwired: 2 in, 1 out]
            n44 = call "FITS - Format FITS Keyword v2 .vi"("Keyword"=w181, "Value"=w178, "Comment"=w180) -> ("Formatted fits entry"=w179:string, "Length of line"=w177:i16)  [unwired: 1 in, 1 out]
          }
          frame "COMMHEAD" {
            n45 = Unbundle By Name(w183) -> ("Comment"=w182:string)
            n46 = call "FITS - Format FITS Keyword v2 .vi"("Keyword"=w187, "Value"=w182, "Comment"=w186) -> ("Formatted fits entry"=w185:string, "Length of line"=w184:i16)  [unwired: 1 in, 1 out]
          }
          frame "COOKBOOK" {
            w190 = "'" ("string")
            n47 = Unbundle By Name(w195) -> ("Cookbook"=w189:string)
            n48 = Concatenate Strings(w190, w189, w190) -> (w188:string)
            n49 = call "FITS - Format FITS Keyword v2 .vi"("Keyword"=w194, "Value"=w188, "Comment"=w193) -> ("Formatted fits entry"=w192:string, "Length of line"=w191:i16)  [unwired: 1 in, 1 out]
          }
          frame "DATATYPE" {
            w198 = "'" ("string")
            n50 = disable-structure shown="Disabled" {
              disable-tunnel: w203 -> [w206 _]
              disable-tunnel: [w204 w220] -> w197
              frame Enabled {
                n51 = Unbundle By Name(w206) -> ("Data Type"=w205:T4)
                n52 = case shown="\"OBSE\"" w205 {
                  tunnel: ["LIVE" "DARK" "FLAT" "CALI" "OBSE" "ABSO" "AURE" "TARG" "OBJE" "HOLE" "OREX" "THRO" "CHIP"] -> w204
                  frame "LIVE", Default {
                  }
                  frame "DARK" {
                  }
                  frame "FLAT" {
                  }
                  frame "CALI" {
                  }
                  frame "OBSE" {
                  }
                  frame "ABSO" {
                  }
                  frame "AURE" {
                  }
                  frame "TARG" {
                  }
                  frame "OBJE" {
                  }
                  frame "HOLE" {
                  }
                  frame "OREX" {
                  }
                  frame "THRO" {
                  }
                  frame "CHIP" {
                  }
                }
              }
              frame Disabled {
                n53 = property on="Data Type" class="Enum (strict)"() -> ("RingText.Text"=w220:string)  [unwired: 2 in, 2 out]
              }
            }
            n54 = Concatenate Strings(w198, w197, w198) -> (w196:string)
            n55 = call "FITS - Format FITS Keyword v2 .vi"("Keyword"=w202, "Value"=w196, "Comment"=w201) -> ("Formatted fits entry"=w200:string, "Length of line"=w199:i16)  [unwired: 1 in, 1 out]
          }
          frame "DATE" {
            n56 = Unbundle By Name(w221) -> ("Date"=w222:string)
            n57 = call "FITS - Format FITS Keyword v2 .vi"("Keyword"=w226, "Value"=w222, "Comment"=w225) -> ("Formatted fits entry"=w224:string, "Length of line"=w223:i16)  [unwired: 1 in, 1 out]
          }
          frame "DATE-OBS" {
            # "FITS standard says that the DATE_OBS keyword is used for \nthe START of the observation"
            n58 = disable-structure shown="Enabled" {
              disable-tunnel: w230 -> [w235 w239]
              disable-tunnel: [w236 w242] -> w229
              disable-tunnel: w227 -> [_ _]
              frame Enabled {
                # "ten isty cas ako vo fits name"
                n59 = Unbundle By Name(w235) -> ("Time Start"=w234:timestamp)
                n60 = Format Date/Time String(time format string (%c)="%Y-%m-%dT%H:%M:%S", seconds (now)=w234) -> (date/time string=w236:string)  [unwired: 1 in]
              }
              frame Disabled {
                # "cas frame1 a zaokruhluje sa na sekundy"
                n61 = Unbundle By Name(w239) -> ("Time Stamp Array"=w240:timestamp[])
                n62 = Index Array(array=w240, index=0) -> (element=w238:timestamp)
                n63 = Format Date/Time String(time format string (%c)="%Y-%m-%dT%H:%M:%S", seconds (now)=w238) -> (date/time string=w242:string)  [unwired: 1 in]
              }
            }
            n64 = call "FITS - Format FITS Keyword v2 .vi"("Keyword"=w233, "Value"=w229, "Comment"=w232) -> ("Formatted fits entry"=w231:string, "Length of line"=w228:i16)  [unwired: 1 in, 1 out]
          }
          frame "DATE-END" {
            n65 = Unbundle By Name(w250) -> ("Time End"=w245:timestamp)
            n66 = Format Date/Time String(time format string (%c)="%Y-%m-%dT%H:%M:%S", seconds (now)=w245) -> (date/time string=w251:string)  [unwired: 1 in]
            n67 = call "FITS - Format FITS Keyword v2 .vi"("Keyword"=w248, "Value"=w251, "Comment"=w249) -> ("Formatted fits entry"=w246:string, "Length of line"=w247:i16)  [unwired: 1 in, 1 out]
          }
          frame "TIME-FR1" {
            n68 = Unbundle By Name(w258) -> ("Time Stamp Array"=w254:timestamp[])
            n69 = Index Array(array=w254, index=0) -> (element=w253:timestamp)
            n70 = Format Date/Time String(time format string (%c)="%H:%M:%S%3u", seconds (now)=w253) -> (date/time string=w261:string)  [unwired: 1 in]
            n71 = call "FITS - Format FITS Keyword v2 .vi"("Keyword"=w260, "Value"=w261, "Comment"=w259) -> ("Formatted fits entry"=w257:string, "Length of line"=w256:i16)  [unwired: 1 in, 1 out]
          }
          frame "TIME-FR2" {
            n72 = Unbundle By Name(w264) -> ("Time Stamp Array"=w269:timestamp[])
            n73 = Index Array(array=w269, index=1) -> (element=w268:timestamp)
            n74 = Format Date/Time String(time format string (%c)="%H:%M:%S%3u", seconds (now)=w268) -> (date/time string=w271:string)  [unwired: 1 in]
            n75 = call "FITS - Format FITS Keyword v2 .vi"("Keyword"=w266, "Value"=w271, "Comment"=w265) -> ("Formatted fits entry"=w263:string, "Length of line"=w262:i16)  [unwired: 1 in, 1 out]
          }
          frame "TIME-FR3" {
            n76 = Unbundle By Name(w276) -> ("Time Stamp Array"=w279:timestamp[])
            n77 = Index Array(array=w279, index=2) -> (element=w278:timestamp)
            n78 = Format Date/Time String(time format string (%c)="%H:%M:%S%3u", seconds (now)=w278) -> (date/time string=w281:string)  [unwired: 1 in]
            n79 = call "FITS - Format FITS Keyword v2 .vi"("Keyword"=w274, "Value"=w281, "Comment"=w275) -> ("Formatted fits entry"=w273:string, "Length of line"=w272:i16)  [unwired: 1 in, 1 out]
          }
          frame "TIME-FR4" {
            n80 = Unbundle By Name(w282) -> ("Time Stamp Array"=w289:timestamp[])
            n81 = Index Array(array=w289, index=3) -> (element=w288:timestamp)
            n82 = Format Date/Time String(time format string (%c)="%H:%M:%S%3u", seconds (now)=w288) -> (date/time string=w291:string)  [unwired: 1 in]
            n83 = call "FITS - Format FITS Keyword v2 .vi"("Keyword"=w284, "Value"=w291, "Comment"=w283) -> ("Formatted fits entry"=w285:string, "Length of line"=w286:i16)  [unwired: 1 in, 1 out]
          }
          frame "DETECTOR" {
            n84 = call "FITS - Format FITS Keyword v2 .vi"("Keyword"=w295, "Value"="'ANDOR NEO CAMERA'", "Comment"=w294) -> ("Formatted fits entry"=w293:string, "Length of line"=w292:i16)  [unwired: 1 in, 1 out]
          }
          frame "DIFFUSER" {
            n85 = Unbundle By Name(w303) -> ("Light Shapping Diffuser"=w300:T3)
            n86 = Build Array("'OUT OF BEAM'", "'IN BEAM'") -> (w301:string[])
            n87 = Index Array(array=w301, index=w300) -> (element=w299:string)
            n88 = call "FITS - Format FITS Keyword v2 .vi"("Keyword"=w306, "Value"=w299, "Comment"=w305) -> ("Formatted fits entry"=w304:string, "Length of line"=w302:i16)  [unwired: 1 in, 1 out]
          }
          frame "EXPTIME" {
            n89 = Unbundle By Name(w313) -> ("Exposure (s)"=w311:dbl)
            n90 = Multiply(x=1000.0, y=w311) -> (x*y=w308:dbl)
            n91 = Format Into String(format string="%_3f", w308) -> (resulting string=w312:string)  [unwired: 2 in, 1 out]
            n92 = call "FITS - Format FITS Keyword v2 .vi"("Keyword"=w316, "Value"=w312, "Comment"=w315) -> ("Formatted fits entry"=w314:string, "Length of line"=w310:i16)  [unwired: 1 in, 1 out]
          }
          frame "EXTEND" {
            n93 = call "FITS - Format FITS Keyword v2 .vi"("Keyword"=w321, "Value"="T", "Comment"=w320) -> ("Formatted fits entry"=w319:string, "Length of line"=w317:i16)  [unwired: 1 in, 1 out]
          }
          frame "FILENAME" {
            w324 = "'" ("string")
            n94 = Unbundle By Name(w325) -> ("File name"=w323:string)
            n95 = Concatenate Strings(w324, w323, w324) -> (w322:string)
            n96 = call "FITS - Format FITS Keyword v2 .vi"("Keyword"=w329, "Value"=w322, "Comment"=w328) -> ("Formatted fits entry"=w327:string, "Length of line"=w326:i16)  [unwired: 1 in, 1 out]
          }
          frame "FILTER" {
            n97 = disable-structure shown="SCMP==COMP, Default" {
              disable-tunnel: ["'HAO Lyot 4-stage'" "'HAO Lyot 5-stage'"] -> w330
              frame condition #0 (active) {
              }
              frame condition #1 {
              }
            }
            n98 = call "FITS - Format FITS Keyword v2 .vi"("Keyword"=w334, "Value"=w330, "Comment"=w333) -> ("Formatted fits entry"=w332:string, "Length of line"=w331:i16)  [unwired: 1 in, 1 out]
          }
          frame "FLC-1" {
            n99 = call "FITS - Format FITS Keyword v2 .vi"("Keyword"=w341, "Value"="'+5.00,-5.00,+5.00,-5.00'", "Comment"=w340) -> ("Formatted fits entry"=w338:string, "Length of line"=w339:i16)  [unwired: 1 in, 1 out]
          }
          frame "FLC-2" {
            n100 = call "FITS - Format FITS Keyword v2 .vi"("Keyword"=w345, "Value"="'+5.00,-5.00,-5.00,+5.00'", "Comment"=w344) -> ("Formatted fits entry"=w343:string, "Length of line"=w342:i16)  [unwired: 1 in, 1 out]
          }
          frame "FOCUS" {
            n101 = Unbundle By Name(w350) -> ("Objective Lens Position (mm)"=w349:T9)
            n102 = Format Into String(format string="%5.2f", w349) -> (resulting string=w354:string)  [unwired: 2 in, 1 out]
            n103 = call "FITS - Format FITS Keyword v2 .vi"("Keyword"=w353, "Value"=w354, "Comment"=w352) -> ("Formatted fits entry"=w351:string, "Length of line"=w348:i16)  [unwired: 1 in, 1 out]
          }
          frame "FW-CALIB" {
            w357 = "'" ("string")
            n104 = disable-structure shown="SCMP==COMP, Default" {
              disable-tunnel: w359 -> [w375 w388]
              disable-tunnel: [w373 w386] -> w356
              frame condition #0 {
                n105 = Unbundle By Name(w375) -> ("SCD Calibration Optics"=w374:T5)
                n106 = Build Array("LP0, I+Q", "LP90, I-Q", "LP45, I+U", "LP135, I-U" ("element"), "LCP, I+V" ("element"), "RCP, I-V" ("element"), "Dark" ("element"), "Clear" ("element"), "N/A" ("element")) -> (w363:string[])
                n107 = Index Array(array=w363, index=w374) -> (element=w373:string)
              }
              frame condition #1 (active) {
                n108 = Unbundle By Name(w388) -> ("COMP-S Calibration Wheel"=w387:T7)
                n109 = Build Array("Dark", "Clear", "Lens", "I+Q" ("element"), "I-Q" ("element"), "I+U" ("element"), "I-U" ("element"), "I+V" ("element"), "I-V" ("element")) -> (w378:string[])
                n110 = Index Array(array=w378, index=w387) -> (element=w386:string)
              }
            }
            n111 = Concatenate Strings(w357, w356, w357) -> (w355:string)
            n112 = call "FITS - Format FITS Keyword v2 .vi"("Keyword"=w362, "Value"=w355, "Comment"=w361) -> ("Formatted fits entry"=w360:string, "Length of line"=w358:i16)  [unwired: 1 in, 1 out]
          }
          frame "FW-WVLNG" {
            n113 = call "SCMP get wave from fw.vi"("FITS Header"=w390) -> ("element"=w389:string)  [unwired: 9 in, 1 out]
            n114 = call "FITS - Format FITS Keyword v2 .vi"("Keyword"=w394, "Value"=w389, "Comment"=w393) -> ("Formatted fits entry"=w392:string, "Length of line"=w391:i16)  [unwired: 1 in, 1 out]
          }
          frame "GCOUNT" {
            n115 = call "FITS - Format FITS Keyword v2 .vi"("Keyword"=w399, "Value"="1", "Comment"=w397) -> ("Formatted fits entry"=w396:string, "Length of line"=w395:i16)  [unwired: 1 in, 1 out]
          }
          frame "INSTRUME" {
            n116 = disable-structure shown="SCMP==SCD" {
              disable-tunnel: ["'COMP-S'" "'SCD'"] -> w400
              frame condition #0 (active) {
              }
              frame condition #1 {
              }
            }
            n117 = call "FITS - Format FITS Keyword v2 .vi"("Keyword"=w404, "Value"=w400, "Comment"=w403) -> ("Formatted fits entry"=w402:string, "Length of line"=w401:i16)  [unwired: 1 in, 1 out]
          }
          frame "LOCATION" {
            n118 = call "FITS - Format FITS Keyword v2 .vi"("Keyword"=w411, "Value"="'LOMNICKY PEAK OBSERVATORY'", "Comment"=w409) -> ("Formatted fits entry"=w410:string, "Length of line"=w408:i16)  [unwired: 1 in, 1 out]
          }
          frame "LEVEL" {
            n119 = call "FITS - Format FITS Keyword v2 .vi"("Keyword"=w415, "Value"="0", "Comment"=w414) -> ("Formatted fits entry"=w413:string, "Length of line"=w412:i16)  [unwired: 1 in, 1 out]
          }
          frame "MODC" {
            n120 = Unbundle By Name(w419) -> ("Mod Cycles"=w418:u16)
            n121 = Format Into String(format string="%d", w418) -> (resulting string=w423:string)  [unwired: 2 in, 1 out]
            n122 = call "FITS - Format FITS Keyword v2 .vi"("Keyword"=w422, "Value"=w423, "Comment"=w421) -> ("Formatted fits entry"=w420:string, "Length of line"=w417:i16)  [unwired: 1 in, 1 out]
          }
          frame "NAXIS" {
            n123 = Equal To 0?(x=w425) -> (x = 0?=w426:bool)
            n124 = case shown="False" w426 {
              tunnel: w430 -> [w433 w440]
              tunnel: w429 -> [w434 w439]
              tunnel: [w432 w438] -> w428
              tunnel: [w431 w437] -> w427
              frame False {
                # "All SCD Images have\n3 dimensions\nx-pixels\ny-pixels\npol state"
                n125 = call "FITS - Format FITS Keyword v2 .vi"("Keyword"=w433, "Value"="3", "Comment"=w434) -> ("Formatted fits entry"=w432:string, "Length of line"=w431:i16)  [unwired: 1 in, 1 out]
              }
              frame True {
                n126 = call "FITS - Format FITS Keyword v2 .vi"("Keyword"=w440, "Value"="0", "Comment"=w439) -> ("Formatted fits entry"=w438:string, "Length of line"=w437:i16)  [unwired: 1 in, 1 out]
              }
            }
          }
          frame "NAXIS1" {
            # "mh maj19 kamera na COMP-S je otocena o 90st\nmh jul19 -aj tak nakoniec netreba rotovat"
            n127 = disable-structure shown="SCMP==SCD" {
              disable-tunnel: [w450 w451] -> w443
              disable-tunnel: w442 -> [w450 w451]
              disable-tunnel: w441 -> [_ _]
              frame condition #0 (active) {
              }
              frame condition #1 {
              }
            }
            n128 = Number To Decimal String(number=w443, width (-)=i16 4) -> (decimal integer string=w444:string)
            n129 = call "FITS - Format FITS Keyword v2 .vi"("Keyword"=w449, "Value"=w444, "Comment"=w448) -> ("Formatted fits entry"=w447:string, "Length of line"=w446:i16)  [unwired: 1 in, 1 out]
          }
          frame "NAXIS2" {
            # "mh maj19 kamera na COMP-S je otocena o 90st\nmh jul19 -aj tak nakoniec netreba rotovat"
            n130 = disable-structure shown="SCMP==SCD" {
              disable-tunnel: [w461 w462] -> w458
              disable-tunnel: w453 -> [w461 w462]
              disable-tunnel: w452 -> [_ _]
              frame condition #0 (active) {
              }
              frame condition #1 {
              }
            }
            n131 = Number To Decimal String(number=w458, width (-)=i16 4) -> (decimal integer string=w459:string)
            n132 = call "FITS - Format FITS Keyword v2 .vi"("Keyword"=w456, "Value"=w459, "Comment"=w457) -> ("Formatted fits entry"=w455:string, "Length of line"=w454:i16)  [unwired: 1 in, 1 out]
          }
          frame "NAXIS3" {
            # "For a \"Snapshot\" NAXIS is 1\nFor cookbook based observations NAXIS is 4\n\nThe SCD modulator produces 4 modulation states\nhereafter know as A,B,C,D."
            n133 = call "FITS - Format FITS Keyword v2 .vi"("Keyword"=w467, "Value"="NAXIS", "Comment"=w466) -> ("Formatted fits entry"=w465:string, "Length of line"=w464:i16)  [unwired: 1 in, 1 out]
          }
          frame "NAXIS4" {
            # "SCD is a single camera instrument"
            n134 = call "FITS - Format FITS Keyword v2 .vi"("Keyword"=w472, "Value"="1", "Comment"=w471) -> ("Formatted fits entry"=w470:string, "Length of line"=w468:i16)  [unwired: 1 in, 1 out]
          }
          frame "NLC-1" {
            n135 = Unbundle By Name(w479) -> ("Tuning Voltages"=w475:dbl[])
            n136 = Index Array(array=w475, index=0) -> (element=w474:dbl)
            n137 = Format Into String(format string="%0.3f", w474) -> (resulting string=w473:string)  [unwired: 2 in, 1 out]
            n138 = call "FITS - Format FITS Keyword v2 .vi"("Keyword"=w482, "Value"=w473, "Comment"=w481) -> ("Formatted fits entry"=w480:string, "Length of line"=w478:i16)  [unwired: 1 in, 1 out]
          }
          frame "NLC-2" {
            n139 = Unbundle By Name(w489) -> ("Tuning Voltages"=w485:dbl[])
            n140 = Index Array(array=w485, index=1) -> (element=w484:dbl)
            n141 = Format Into String(format string="%0.3f", w484) -> (resulting string=w483:string)  [unwired: 2 in, 1 out]
            n142 = call "FITS - Format FITS Keyword v2 .vi"("Keyword"=w492, "Value"=w483, "Comment"=w491) -> ("Formatted fits entry"=w490:string, "Length of line"=w488:i16)  [unwired: 1 in, 1 out]
          }
          frame "NLC-3" {
            n143 = Unbundle By Name(w499) -> ("Tuning Voltages"=w495:dbl[])
            n144 = Index Array(array=w495, index=2) -> (element=w494:dbl)
            n145 = Format Into String(format string="%0.3f", w494) -> (resulting string=w493:string)  [unwired: 2 in, 1 out]
            n146 = call "FITS - Format FITS Keyword v2 .vi"("Keyword"=w502, "Value"=w493, "Comment"=w501) -> ("Formatted fits entry"=w500:string, "Length of line"=w498:i16)  [unwired: 1 in, 1 out]
          }
          frame "NLC-4" {
            n147 = Unbundle By Name(w509) -> ("Tuning Voltages"=w505:dbl[])
            n148 = Index Array(array=w505, index=3) -> (element=w504:dbl)
            n149 = Format Into String(format string="%0.3f", w504) -> (resulting string=w503:string)  [unwired: 2 in, 1 out]
            n150 = call "FITS - Format FITS Keyword v2 .vi"("Keyword"=w512, "Value"=w503, "Comment"=w511) -> ("Formatted fits entry"=w510:string, "Length of line"=w508:i16)  [unwired: 1 in, 1 out]
          }
          frame "NLC-5" {
            n151 = Unbundle By Name(w519) -> ("Tuning Voltages"=w515:dbl[])
            n152 = Index Array(array=w515, index=4) -> (element=w514:dbl)
            n153 = Format Into String(format string="%0.3f", w514) -> (resulting string=w513:string)  [unwired: 2 in, 1 out]
            n154 = call "FITS - Format FITS Keyword v2 .vi"("Keyword"=w522, "Value"=w513, "Comment"=w521) -> ("Formatted fits entry"=w520:string, "Length of line"=w518:i16)  [unwired: 1 in, 1 out]
          }
          frame "OBSERVER" {
            w525 = "'" ("string")
            n155 = Unbundle By Name(w526) -> ("Observer"=w524:string)
            n156 = Concatenate Strings(w525, w524, w525) -> (w523:string)
            n157 = call "FITS - Format FITS Keyword v2 .vi"("Keyword"=w530, "Value"=w523, "Comment"=w529) -> ("Formatted fits entry"=w528:string, "Length of line"=w527:i16)  [unwired: 1 in, 1 out]
          }
          frame "OBS_PROG" {
            w533 = "'" ("string")
            n158 = Unbundle By Name(w536) -> ("Comment"=w532:string)
            n159 = Concatenate Strings(w533, w532, w533) -> (w531:string)
            n160 = call "FITS - Format FITS Keyword v2 .vi"("Keyword"=w538, "Value"=w531, "Comment"=w537) -> ("Formatted fits entry"=w534:string, "Length of line"=w535:i16)  [unwired: 1 in, 1 out]
          }
          frame "OCC-SIZE" {
            n161 = Unbundle By Name(w542) -> ("Occulter size"=w541:dbl)
            n162 = Format Into String(format string="%5.2f", w541) -> (resulting string=w546:string)  [unwired: 2 in, 1 out]
            n163 = call "FITS - Format FITS Keyword v2 .vi"("Keyword"=w545, "Value"=w546, "Comment"=w544) -> ("Formatted fits entry"=w543:string, "Length of line"=w540:i16)  [unwired: 1 in, 1 out]
          }
          frame "ORIGIN" {
            n164 = call "FITS - Format FITS Keyword v2 .vi"("Keyword"=w551, "Value"="'AISAS'", "Comment"=w550) -> ("Formatted fits entry"=w549:string, "Length of line"=w548:i16)  [unwired: 1 in, 1 out]
          }
          frame "PCOUNT" {
            n165 = call "FITS - Format FITS Keyword v2 .vi"("Keyword"=w556, "Value"="0", "Comment"=w554) -> ("Formatted fits entry"=w553:string, "Length of line"=w552:i16)  [unwired: 1 in, 1 out]
          }
          frame "ROTPOS" {
            n166 = Unbundle By Name(w564) -> ("FOV Rotation (deg)"=w563:dbl)
            n167 = Format Into String(format string="%5.1f", w563) -> (resulting string=w562:string)  [unwired: 2 in, 1 out]
            n168 = call "FITS - Format FITS Keyword v2 .vi"("Keyword"=w560, "Value"=w562, "Comment"=w561) -> ("Formatted fits entry"=w559:string, "Length of line"=w558:i16)  [unwired: 1 in, 1 out]
          }
          frame "APERTURE" {
            n169 = Unbundle By Name(w577) -> ("Abso Aperture"=w568:dbl, "Nominal Aperture"=w567:dbl, "Data Type"=w570:T4)
            n170 = Equal?(x=w570, y=FITS_Data_type."ABSO") -> (x = y?=w569:bool)
            n171 = Select(t=w568, s=w569, f=w567) -> (s? t:f=w566:dbl)
            n172 = Format Into String(format string="%6.1f", w566) -> (resulting string=w576:string)  [unwired: 2 in, 1 out]
            n173 = call "FITS - Format FITS Keyword v2 .vi"("Keyword"=w574, "Value"=w576, "Comment"=w575) -> ("Formatted fits entry"=w573:string, "Length of line"=w572:i16)  [unwired: 1 in, 1 out]
          }
          frame "SIMPLE" {
            # "FITS Standard Keyword (scott is not sure what it means)"
            n174 = call "FITS - Format FITS Keyword v2 .vi"("Keyword"=w582, "Value"="T", "Comment"=w581) -> ("Formatted fits entry"=w580:string, "Length of line"=w578:i16)  [unwired: 1 in, 1 out]
          }
          frame "TELESCOP" {
            n175 = call "FITS - Format FITS Keyword v2 .vi"("Keyword"=w587, "Value"="'ZEISS 200/3000 CORONAGRAPH'", "Comment"=w586) -> ("Formatted fits entry"=w585:string, "Length of line"=w584:i16)  [unwired: 1 in, 1 out]
          }
          frame "TIMESYS" {
            n176 = call "FITS - Format FITS Keyword v2 .vi"("Keyword"=w591, "Value"="'UTC'", "Comment"=w590) -> ("Formatted fits entry"=w589:string, "Length of line"=w588:i16)  [unwired: 1 in, 1 out]
          }
          frame "TUNEDLAY" {
            n177 = Unbundle By Name(w594) -> ("Tuning Delay (ms)"=w600:dbl)
            n178 = Format Into String(format string="%d", w600) -> (resulting string=w598:string)  [unwired: 2 in, 1 out]
            n179 = call "FITS - Format FITS Keyword v2 .vi"("Keyword"=w597, "Value"=w598, "Comment"=w596) -> ("Formatted fits entry"=w595:string, "Length of line"=w593:i16)  [unwired: 1 in, 1 out]
          }
          frame "WAVELENG" {
            n180 = Unbundle By Name(w605) -> ("Wavelength (nm)"=w604:dbl)
            n181 = Format Into String(format string="%0.3f", w604) -> (resulting string=w602:string)  [unwired: 2 in, 1 out]
            n182 = call "FITS - Format FITS Keyword v2 .vi"("Keyword"=w608, "Value"=w602, "Comment"=w607) -> ("Formatted fits entry"=w606:string, "Length of line"=w601:i16)  [unwired: 1 in, 1 out]
          }
          frame "XTENSION" {
            n183 = call "FITS - Format FITS Keyword v2 .vi"("Keyword"=w613, "Value"="'IMAGE'", "Comment"=w612) -> ("Formatted fits entry"=w611:string, "Length of line"=w609:i16)  [unwired: 1 in, 1 out]
          }
          frame "XPOSURE" {
            n184 = Unbundle By Name(w616) -> ("Acc Exposure (s)"=w615:dbl)
            n185 = Format Into String(format string="%_3f", w615) -> (resulting string=w621:string)  [unwired: 2 in, 1 out]
            n186 = call "FITS - Format FITS Keyword v2 .vi"("Keyword"=w620, "Value"=w621, "Comment"=w619) -> ("Formatted fits entry"=w618:string, "Length of line"=w617:i16)  [unwired: 1 in, 1 out]
          }
        }
      }
      n187 = Array Size(array=w22) -> (size(s)=w18:i32)
      "Header Rows" <- w18
      n188 = Divide(x=23040, y=80) -> (x/y=w19:dbl)
      n189 = Subtract(x=w19, y=w18) -> (x-y=w17:dbl)
      n190 = Decrement(x=w17) -> (x-1=w16:dbl)
      "Required COMMENT Rows" <- w16
      n191 = Format Into String(format string="COMMENT%73s", "") -> (resulting string=w25:string)  [unwired: 2 in, 1 out]
      n192 = for {
        N: w16 -> [_]
        tunnel: w25 -> [w42]
        tunnel: [w42] -> w24 mode=indexing
      }
      n193 = Format Into String(format string="END%77s", "") -> (resulting string=w29:string)  [unwired: 2 in, 1 out]
      n194 = Build Array (concatenate)(w22, w24, w29) -> (w31:string[])
      "FITS Header" <- w31
      n195 = for {
        tunnel: w31 -> [w44] mode=indexing
        shift-right: [w45] -> w28
        shift-left: "" -> [w43]
        n196 = Concatenate Strings(w43, w44) -> (w45:string)
      }
      "23040 Byte Header" <- w28
      n197 = String Length(string=w28) -> (length=→"final header byte length":i32)
    }
    frame Error {
    }
  }
  "error out" <- w5
